vi "Set Plot Color (WDTWFGraph).vi"(7 "Size (24)":i32=24, 8 "error in (no error)":errorcluster, 10 "Active Plot":i32, 11 "WFGraph (WDT) in":refnum<vi>) -> (0 "error out":errorcluster, 2 "Active Plot":i32, 3 "WFGraph (WDT) out":refnum<vi>)   [LabVIEW 2019, in "Instrument.Lockin.lvlib" / "Instrument UI.Lockin.lvclass"]
uses:
  Instrument UI.Lockin.lvclass
  <vilib>/PRIrvin/Graph Utilities/graph_utilities.lvclass
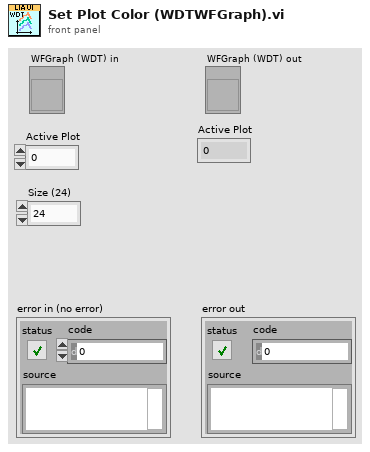
[diagram p1: front panel]
types:
  T1 = enum16{"CET-C1", "CET-C1s", "CET-C2", "CET-C2s", "CET-C3", "CET-C3s", "CET-C4", "CET-C4s", "CET-C5", "CET-C5s", "CET-C6", "CET-C6s", "CET-C7", "CET-C7s", "CET-CBC1", "CET-CBC2", "CET-CBD1", "CET-CBL1", "CET-CBL2", "CET-D01", "CET-D01A", "CET-D02", "CET-D03", "CET-D04", "CET-D06", "CET-D07", "CET-D08", "CET-D09", "CET-D10", "CET-D11", "CET-D12", "CET-D13", "CET-I1", "CET-I2", "CET-I3", "CET-L01", "CET-L02", "CET-L03", "CET-L04", "CET-L05", "CET-L06", "CET-L07", "CET-L08", "CET-L09", "CET-L10", "CET-L11", "CET-L12", "CET-L13", "CET-L14", "CET-L15", "CET-L16", "CET-L17", "CET-L18", "CET-L19", "CET-L20", "CET-R1", "CET-R2", "CET-R3", "CET-R4"}
  T2 = enum16{"Inferno", "Kindlmann", "Plasma", "Viridis", "LevyLab2010", "ColorCET...", "Custom..."}
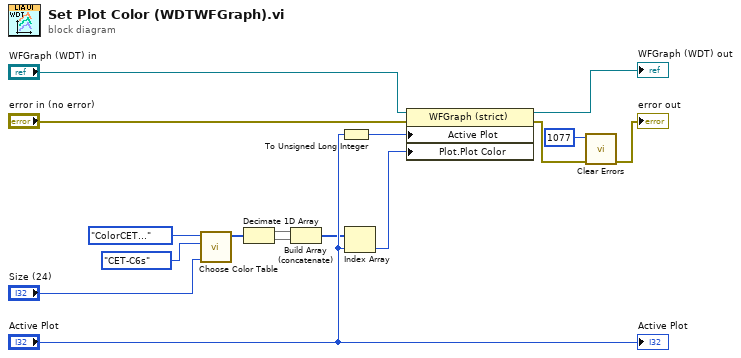
[diagram p0: block diagram]
diagram:
  n1 = call <vilib>:"Choose Color Table.vi"("Size (256)"="Size (24)", "ColorCET"=T1."CET-C6s", "Color Map"=T2."ColorCET...") -> ("Color Table"=w6:u32[])  [unwired: 5 in, 3 out]
  n2 = Decimate 1D Array(w6) -> (w11:u32[], w10:u32[])
  n3 = Build Array (concatenate)(w11, w10) -> (w3:u32[])
  n4 = To Unsigned Long Integer(number="Active Plot") -> (unsigned 32bit integer=w12:u32)
  n5 = Index Array(array=w3, index="Active Plot") -> (element=w2:u32)
  n6 = property on="Property Node" class="WFGraph (strict)"(reference="WFGraph (WDT) in", error in="error in (no error)", "Active Plot"=w12, "Plot.Plot Color"=w2) -> (reference out=→"WFGraph (WDT) out":refnum<vi>, error out=w1:errorcluster)
  n7 = call <vilib>:"Clear Errors.vi"("error in (no error)"=w1, "specific error code to clear (0: all)"=1077) -> ("error out"=→"error out":errorcluster)  [unwired: 4 in, 1 out]
  "Active Plot" <- "Active Plot"
